vi "Apply Voltage.vi"(8 "error in (no error)":errorcluster, 11 "Tool Rectangle in":refnum<class "Tool Rectangle.lvclass">) -> (0 "error out":errorcluster, 3 "Tool Rectangle out":refnum<class "Tool Rectangle.lvclass">)   [LabVIEW 2019, in "Tool Rectangle.lvclass"]
uses:
  Tool Rectangle.lvclass
  Settings/ObjectSettings/ObjectSettings.lvclass/ObjectSettings.ctl
  Settings/Rectangle Settings/Rectangle Settings.lvclass
  C:/Users/Albro/Documents/GitHub/AFM-Lithography/lvsrc/Classes/Settings/ObjectSettings/ObjectSettings.lvclass
  Settings/ObjectSettings/ObjectSettings.lvclass
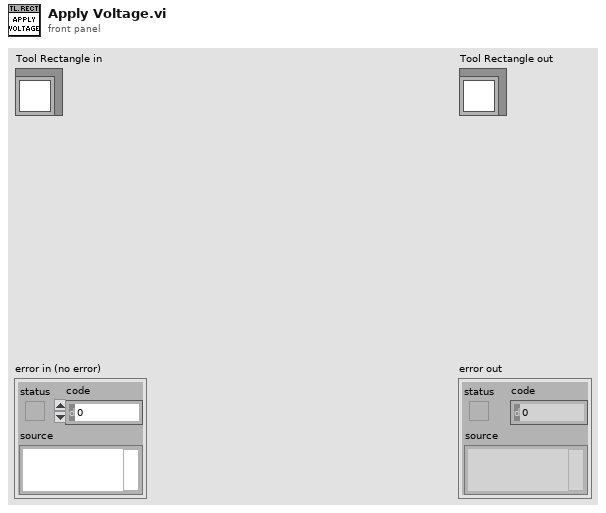
[diagram p1: front panel]
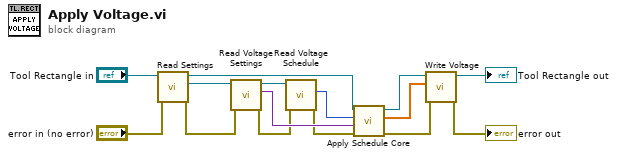
[diagram p0: block diagram]
diagram:
  n1 = call-dynamic "Read Settings.vi"("error in (no error)"="error in (no error)", "Tool Rectangle in"="Tool Rectangle in") -> ("error out"=w4:errorcluster, "Rectangle Settings.lvclass"=w3:refnum<class "Rectangle Settings.lvclass">, "Tool Rectangle out"=w2:refnum<class "Tool Rectangle.lvclass">)  [unwired: 7 in]
  n2 = call "Read Voltage Settings.vi"("error in (no error)"=w4, "ObjectSettings in"=w3) -> ("error out"=w9:errorcluster, "Settings"=w14:variant, "ObjectSettings out"=w15:refnum<class "Rectangle Settings.lvclass">)  [unwired: 7 in]
  n3 = call "Read Voltage Schedule.vi"("error in (no error)"=w9, "ObjectSettings in"=w15) -> ("error out"=w12:errorcluster, "Schedule"=w13:u16)  [unwired: 7 in, 1 out]
  n4 = call-dynamic "Apply Schedule Core.vi"("error in (no error)"=w12, "Settings"=w14, "Schedule"=w13, "Tool Object in"=w2) -> ("error out"=w11:errorcluster, "Schedule Array"=w8:dbl[], "Tool Object out"=w10:refnum<class "Tool Rectangle.lvclass">)  [unwired: 5 in]
  n5 = call-dynamic "Write Voltage.vi"("error in (no error)"=w11, "Voltage"=w8, "Tool Object in"=w10) -> ("error out"=→"error out":errorcluster, "Tool Object out"=→"Tool Rectangle out":refnum<class "Tool Rectangle.lvclass">)  [unwired: 7 in]
